vi "Servo.vi"() -> ()   [LabVIEW 2021]
uses:
  <vilib>/MakerHub/LINX/Public/Utilities/Open Serial.vi
  <vilib>/MakerHub/LINX/Public/Sensors/Motion/Servo/Servo Open One Channel.vi
  <vilib>/MakerHub/LINX/Public/Sensors/Motion/Servo/Servo Set Pulse Width One Channel.vi
  <vilib>/MakerHub/LINX/Public/Sensors/Motion/Servo/Servo Close One Channel.vi
  <vilib>/MakerHub/LINX/LMH-LINX.lvlib
  <vilib>/MakerHub/LINX/Public/Sensors/Motion/Servo/Servo.lvlib
  <vilib>/Analysis/NI_AALPro.lvlib
panel:
  in  "Servo Angle":dbl(knob) min=0.0 max=165.0 step=5.0 scale=0.0..180.0
  in  "stop program":bool
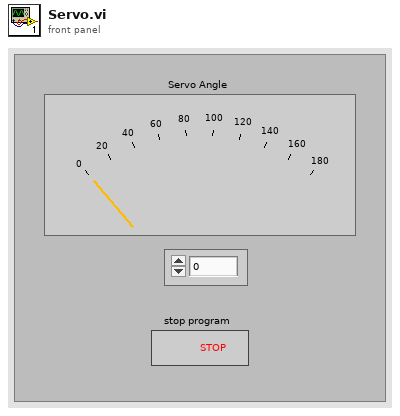
[diagram p1: front panel]
types:
  T1 = typedef "LMH-LINX.lvlib/LINX Ref.ctl" = cluster{"IO":T2, "Interface":T3, "LINX Device Config":T4}
  T2 = typedef "LMH-LINX.lvlib/Platform.ctl" = enum16{"Remote", "Local"}
  T3 = typedef "LMH-LINX.lvlib/Interface.ctl" = enum16{"Serial", "TCP"}
  T4 = typedef "LMH-LINX.lvlib/Device.lvlib/LINX Device Config.ctl" = cluster{"Interface":T3, "COM Port":refnum<visa-resource-name>, "TCP Configuration":T5, "Device Family":u8, "Device ID":u8, "Device Name":string, "TCP Ref":refnum<k5>, "Channels":T6}
  T5 = typedef "LMH-LINX.lvlib/Device.lvlib/TCP Config.ctl" = cluster{"IP Address":string, "Port":u16}
  T6 = typedef "LMH-LINX.lvlib/Channels.ctl" = cluster{"DI":u8[], "DO":u8[], "AI":u8[], "AO":u8[], "PWM":u8[], "QE":u8[], "UART":u8[], "I2C 2":u8[], "SPI":u8[], "CAN":u8[], "Servo":u8[], "AI Ref (V)":dbl, "AI Resolution (Bits)":u8, "AO Ref (V)":dbl, "AO Resolution (Bits)":u8}
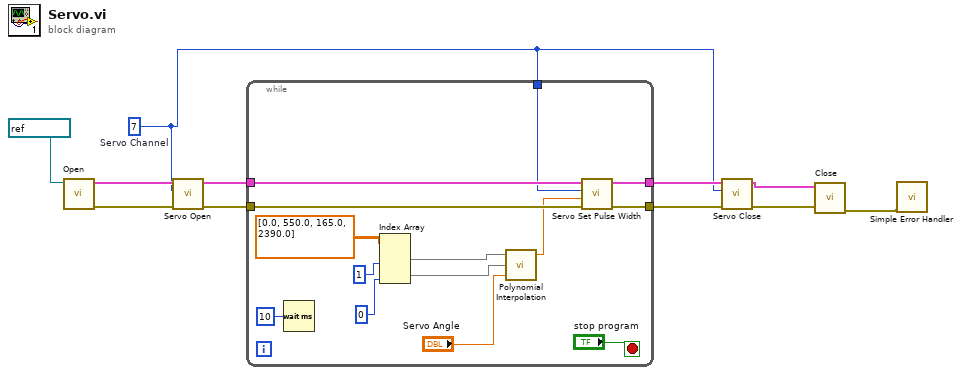
[diagram p0: block diagram]
diagram:
  w1 = 7  # Servo Channel
  n1 = call-poly <vilib>:"Open.vi"("Serial Port"=refnum<visa-resource-name> "COM9") -> ("Error Out"=w7:errorcluster, "LINX Resource"=w8:T1)  [unwired: 8 in, 1 out]
  n2 = call-poly <vilib>:"Servo Open.vi"("Error In"=w7, "Servo Channel"=w1, "LINX Resource"=w8) -> ("Error Out"=w6:errorcluster, "LINX Resource"=w9:T1)  [unwired: 7 in]
  n3 = while {
    tunnel: [w25] -> w10
    tunnel: w9 -> [w24]
    tunnel: w6 -> [w23]
    tunnel: [w22] -> w5
    tunnel: w1 -> [w19]
    stop <- "stop program" stop-if-true
    n4 = Wait (ms)(milliseconds to wait=u32 10) -> ()  [unwired: 1 out]
    n5 = Index Array(array=dbl[][] [[0.0, 550.0], [165.0, 2390.0]], index (col) #1=1 ("disabled index (col)"), index (col) #2=0 ("index (col)")) -> (element #1=w16:dbl[], element #2=w15:dbl[])  [unwired: 2 in]
    n6 = call <vilib>:"Polynomial Interpolation.vi"("x value"="Servo Angle", "X"=w15, "Y"=w16) -> ("interpolation value"=w18:dbl)  [unwired: 2 out]
    n7 = call-poly <vilib>:"Servo Set Pulse Width.vi"("Error In"=w23, "Pulse Width (uS)"=w18, "Servo Channel"=w19, "LINX Resource"=w24) -> ("Error Out"=w22:errorcluster, "LINX Resource"=w25:T1)  [unwired: 6 in]
  }
  n8 = call-poly <vilib>:"Servo Close.vi"("Error In"=w5, "Servo Channel"=w1, "LINX Resource"=w10) -> ("Error Out"=w4:errorcluster, "LINX Resource"=w11:T1)  [unwired: 7 in]
  n9 = call <vilib>:"Close.vi"("Error In"=w4, "LINX Resource"=w11) -> ("Error Out"=w3:errorcluster)  [unwired: 9 in]
  n10 = call <vilib>:"Simple Error Handler.vi"("error in (no error)"=w3) -> ()  [unwired: 4 in, 5 out]
